vi "test VIT Verify AND Parameterized.vi"(8 "error in":errorcluster, 11 "Testing Approval Tests in":refnum<class "VITester Extension Tests.lvclass">) -> (0 "error out":errorcluster, 3 "Testing Approval Tests out":refnum<class "VITester Extension Tests.lvclass">)   [LabVIEW 2026, in "VITester Extension Tests.lvclass"]
uses:
  VITester Extension Tests.lvclass
  VITester Extension Tests.lvclass/VITester Extension Tests.ctl
  Source/Extensions/VITester.Extension/VITester.Extension.lvlib
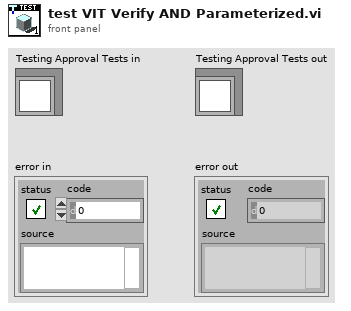
[diagram p1: front panel]
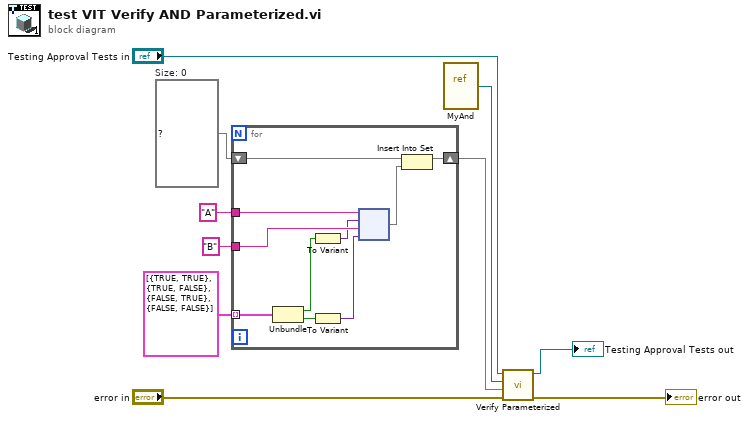
[diagram p0: block diagram]
diagram:
  w3 = set{map{string, variant}} {}  # Size: 0
  n1 = for {
    tunnel: "A" -> [w20]
    tunnel: cluster{bool, bool}[] [{TRUE, TRUE}, {TRUE, FALSE}, {FALSE, TRUE}, {FALSE, FALSE}] -> [w18] mode=indexing
    tunnel: "B" -> [w19]
    shift-right: [w12] -> w2
    shift-left: w3 -> [w11]
    n2 = Unbundle(w18) -> (w17:bool, w16:bool)
    n3 = To Variant(anything=w17) -> (Variant=w14:variant)
    n4 = To Variant(anything=w16) -> (Variant=w13:variant)
    n5 = node(w20, w14, w19, w13) -> (w15:map{string, variant})
    n6 = Insert Into Set(10:w15, 11:w11) -> (3:w12:set{map{string, variant}})  [unwired: 1 out]
  }
  n7 = vi-ref "MyAnd.vi"() -> (w1:refnum<vi>)
  n8 = call "Verify Parameterized.vi"("error in"="error in", "Set of ctl label -> value var"=w2, "VI in"=w1, "TestCase in"="Testing Approval Tests in") -> ("error out"=→"error out":errorcluster, "TestCase out"=→"Testing Approval Tests out":refnum<class "VITester Extension Tests.lvclass">)  [unwired: 6 in]
